vi "conv10toM (SubVI).vi"(8 "max":i16=256, 10 "Base":i16, 11 "Input":i16) -> (3 "Array":u8[](array[numeric]))   [LabVIEW 2017]
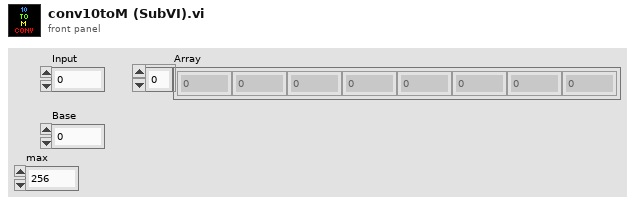
[diagram p1: front panel]
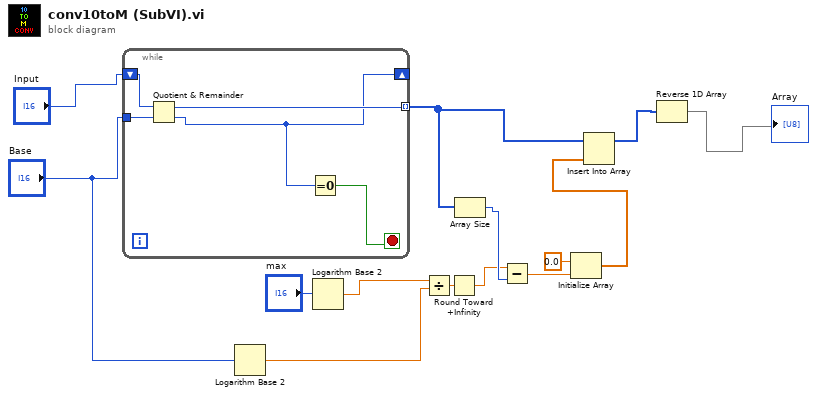
[diagram p0: block diagram]
diagram:
  n1 = while {
    tunnel: "Base" -> [w19]
    tunnel: [w18] -> w7 mode=indexing
    shift-right: [w16] -> _
    shift-left: "Input" -> [w17]
    stop <- w15 stop-if-true
    n2 = Quotient & Remainder(x=w17, y=w19) -> (x-y*floor(x/y)=w18:i16, floor(x/y)=w16:i16)
    n3 = Equal To 0?(x=w16) -> (x = 0?=w15:bool)
  }
  n4 = Logarithm Base 2(1:"Base") -> (0:w9:dbl)
  n5 = Logarithm Base 2(1:"max") -> (0:w3:dbl)
  n6 = Divide(x=w3, y=w9) -> (x/y=w1:dbl)
  n7 = Round Toward +Infinity(x=w1) -> (ceil(x): smallest int >= x=w2:dbl)
  n8 = Array Size(array=w7) -> (size(s)=w13:i32)
  n9 = Subtract(x=w2, y=w13) -> (x-y=w12:dbl)
  n10 = Initialize Array(0.0 ("element"), w12) -> (w6:dbl[])
  n11 = Insert Into Array(array=w7, new element=w6) -> (w5:i16[])  [unwired: 1 in]
  n12 = Reverse 1D Array(array=w5) -> (reversed array=→"Array":i16[])
